vi "io.interface.serial.vi"(0 "IoConf in":T1={"ADDR"=0, "Label"="", "Type"=enum."DI", "Mode"=enum."RIO", "Value"="", "Tags"="", "calibration"=[]} {"calibration"."Y" format="%#.3f"; "calibration"."X" format="%#.3f"; "ADDR" format="%04d"}, 1 "Caller":string, 5 "Output State":variant, 7 "record filename.* (disabled if empty)":string, 9 "current time":timestamp, 11 "error in (no error)":errorcluster, 12 "Save to IO Reg(T)":bool=TRUE) -> (3 "DI":bool[](array[boolean]), 4 "IoConf out":T1={"ADDR"=0, "Label"="", "Type"=enum."DI", "Mode"=enum."RIO", "Value"="", "Tags"="", "calibration"=[]} {"calibration"."Y" format="%#.3f"; "calibration"."X" format="%#.3f"; "ADDR" format="%04d"}, 6 "IN (calib)":dbl, 10 "IN (uncalib)":u16, 14 "Operation Time ms":u32, 15 "error out":errorcluster)   [LabVIEW 2024]
uses:
  controls/IONode.ctl
  controls/type.address.ctl
  controls/enum.io.type.ctl
  controls/enum.io.mode.ctl
  controls/typeXyPoint.ctl
  controls/enum.io-interface.ctl
  controls/enumVarCtrlIO.ctl
  controls/cluster-com-log.ctl
  controls/enum-com-log.ctl
  Polymorphics/io.command-builder.DO.vi
  Polymorphics/io.command-builder.AI.vi
  Polymorphics/io.command-builder.DI.vi
  globals/globals-engine.vi
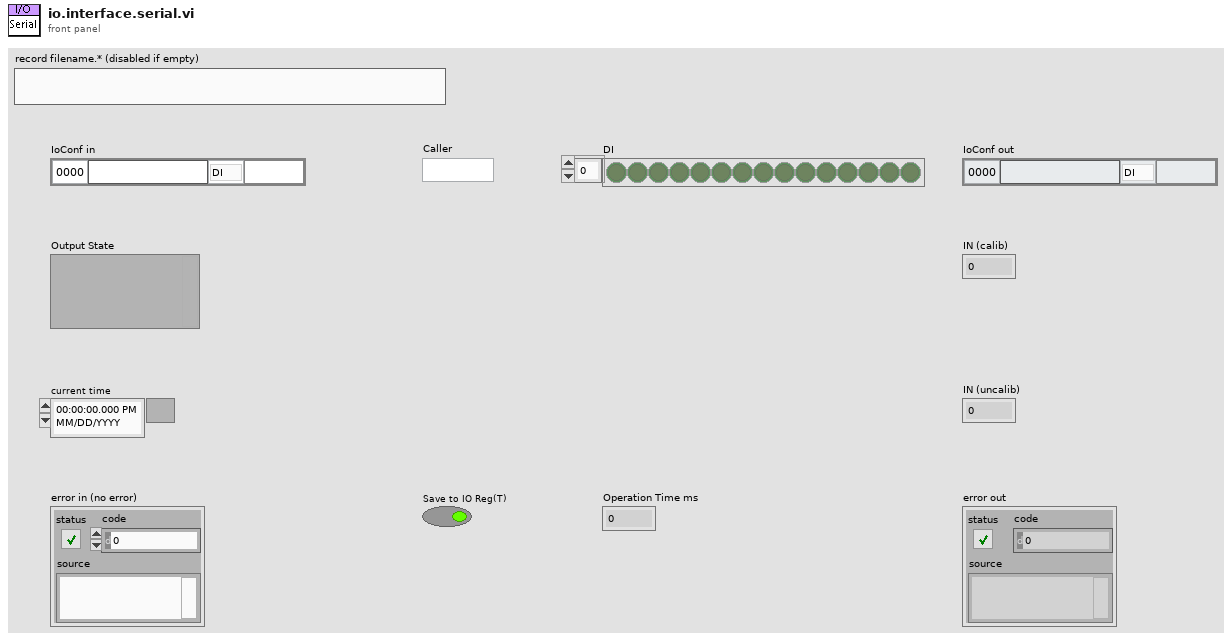
[diagram p1: front panel]
types:
  T1 = typedef "IONode.ctl" = cluster{"ADDR":T2, "Label":string, "Type":T3, "Mode":T4, "Value":string, "Tags":string, "calibration":T5[]}
  T2 = typedef "type.address.ctl" = u16
  T3 = typedef "enum.io.type.ctl" = enum16{"Type", "DI", "DO", "AI", "AO", "VL", "BUF"}
  T4 = typedef "enum.io.mode.ctl" = enum16{"Mode", "RIO", "SIM"}
  T5 = typedef "typeXyPoint.ctl" = cluster{"X":dbl, "Y":dbl}
  T6 = typedef "enum.io-interface.ctl" = enum16{"IO_VISA_WR-RD", "IO_VISA_OPEN", "IO_VISA_CLOSE", "IO_VISA_CLEAR"}
  T7 = typedef "enumVarCtrlIO.ctl" = enum16{"IO Get By Key", "IO List Configs", "IO Add By Key", "IO Modify Value By Key", "IO Modify Calib By Key", "IO Modify ADDR By Key", "IO Modify Mode By Key", "IO Modify Type By Key", "IO Modify Name By Key", "IO Remove By Key", "IO Remove All"}
  T8 = typedef "typeEnv.ctl" = enum16{"ENV.PRODUCTION", "ENV.TEST.NO-HW", "ENV.TEST.SINGLE-01", "ENV.TEST.SINGLE-02", "ENV.TEST.SINGLE-02 AI 0", "ENV.TEST.SINGLE-03"}
  T9 = typedef "cluster-com-log.ctl" = cluster{"Caller":string, "IOnode":T1, "error":errorcluster, "dports":bool[], "AIN (calib)":dbl, "AIN (raw)":u16, "Times Stamp":timestamp, "Record File Path":path, "Visa Data":string}
  T10 = typedef "enum-com-log.ctl" = enum16{"REC.NO_OP", "REC.INIT", "REC.EXIT", "REC.SERIAL", "REC.IO", "REC.FETCH", "REC.OPEN-FILE", "REC.REOPEN-FILE"}
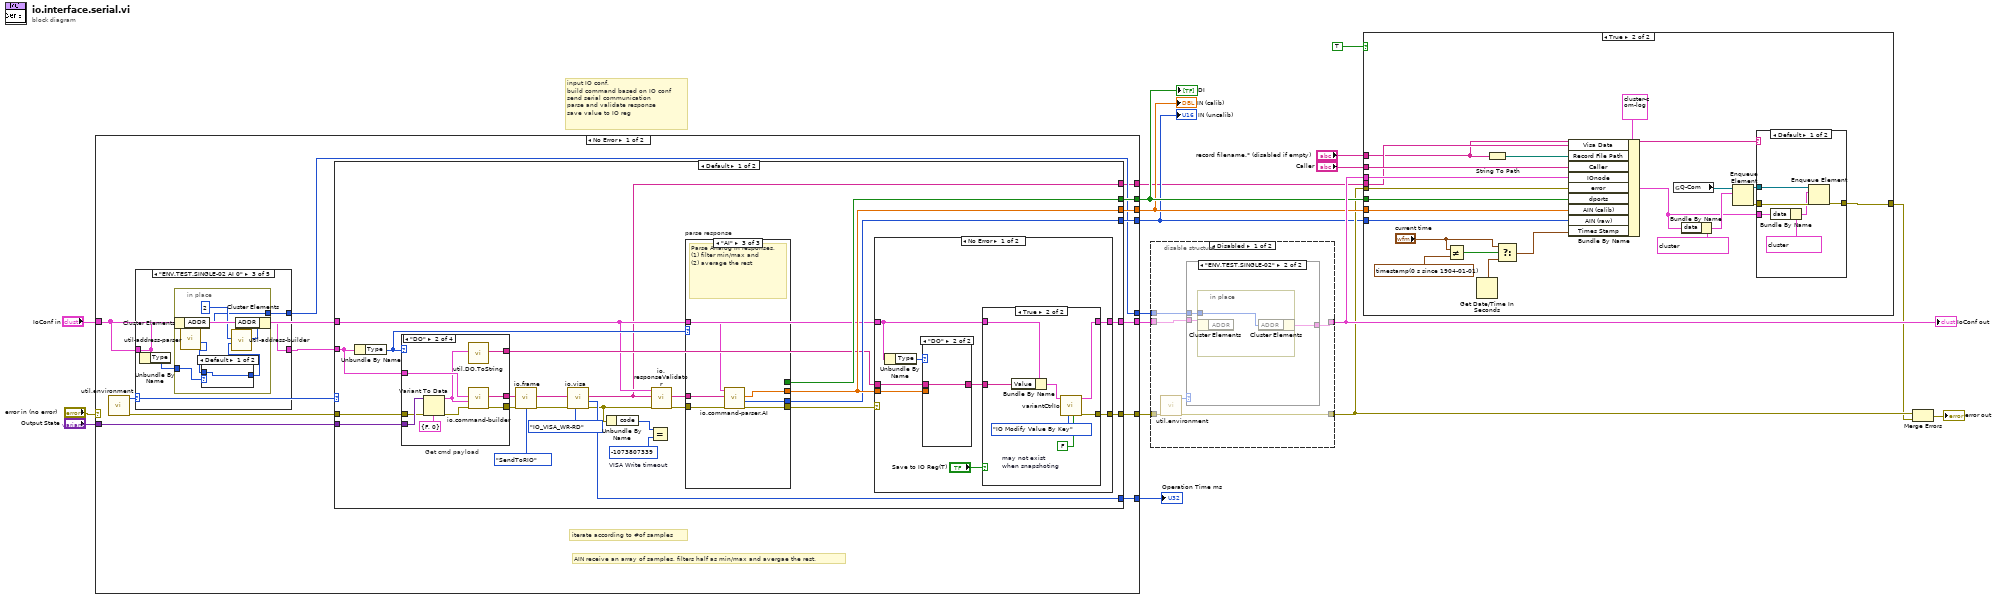
[diagram p0: block diagram]
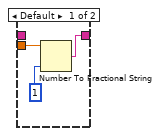
[diagram p6: hidden frame]
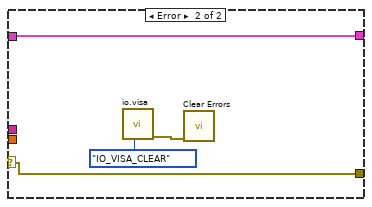
[diagram p8: hidden frame]
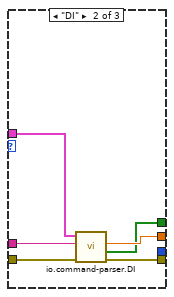
[diagram p10: hidden frame]
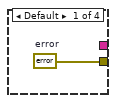
[diagram p11: hidden frame]
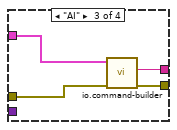
[diagram p12: hidden frame]
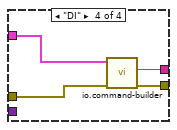
[diagram p13: hidden frame]
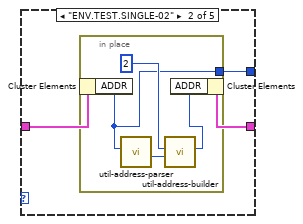
[diagram p16: hidden frame]
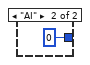
[diagram p17: hidden frame]
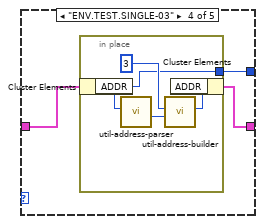
[diagram p18: hidden frame]
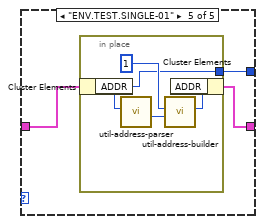
[diagram p19: hidden frame]
diagram:
  # "input IO conf, \nbuild command based on IO conf\nsend serial communication\nparse and validate response\nsave value to IO reg"
  n1 = case shown="No Error" "error in (no error)" {
    selector: "error in (no error)" -> [_ w148]
    tunnel: [w31 _] -> w18
    tunnel: [w30 w148] -> w14
    tunnel: [w29 _] -> w7
    tunnel: [w28 _] -> w4
    tunnel: [w27 _] -> w8
    tunnel: [w26 w147] -> w13
    tunnel: "Output State" -> [w25 _]
    tunnel: "IoConf in" -> [w20 w147]
    tunnel: [w22 _] -> w12
    tunnel: [w19 _] -> w1
    frame No Error {
      # "AIN receive an array of samples, filters half as min/max and avergae the rest."
      # "iterate according to #of samples"
      n2 = call "util.environment.vi"() -> ("error out"=w24:errorcluster, "ENV out"=w21:T8)  [unwired: 10 in]
      n3 = case shown="\"ENV.TEST.SINGLE-02 AI 0\"" w21 {
        tunnel: [w113 w115 w124 w134 w141] -> w23
        tunnel: w20 -> [w113 w116 w122 w135 w142]
        tunnel: [_ w114 w123 w133 w140] -> w22
        frame Default {
        }
        frame "ENV.TEST.SINGLE-02" {
          n4 = in-place {
            in-place-border: [w117] -> w114
            n5 = in-place-cluster #1(w116) -> ("ADDR"=w117:T2)
            n6 = call "util-address-parser.vi"("ADDR 2"=w117) -> ("Channel"=w120:u8)  [unwired: 9 in, 1 out]
            n7 = call "util-address-builder.vi"("Channel"=w120, "Device"=T2 2 ("ADDR")) -> ("ADDR"=w119:T2)  [unwired: 9 in]
            n8 = in-place-cluster #1("ADDR"=w119) -> (w115:T1)
          }
        }
        frame "ENV.TEST.SINGLE-02 AI 0" {
          n9 = Unbundle By Name(w122) -> ("Type"=w121:T3)
          n10 = in-place {
            in-place-border: [w128] -> w123
            in-place-border: w121 -> [w127]
            n11 = in-place-cluster #2(w122) -> ("ADDR"=w128:T2)
            n12 = call "util-address-parser.vi"("ADDR 2"=w128) -> ("Channel"=w126:u8)  [unwired: 9 in, 1 out]
            n13 = case shown="Default" w127 {
              tunnel: [w131 u8 0 ("Channel")] -> w125
              tunnel: w126 -> [w131 _]
              frame Default {
              }
              frame "AI" {
              }
            }
            n14 = call "util-address-builder.vi"("Channel"=w125, "Device"=T2 2 ("ADDR")) -> ("ADDR"=w130:T2)  [unwired: 9 in]
            n15 = in-place-cluster #2("ADDR"=w130) -> (w124:T1)
          }
        }
        frame "ENV.TEST.SINGLE-03" {
          n16 = in-place {
            in-place-border: [w136] -> w133
            n17 = in-place-cluster #3(w135) -> ("ADDR"=w136:T2)
            n18 = call "util-address-parser.vi"("ADDR 2"=w136) -> ("Channel"=w139:u8)  [unwired: 9 in, 1 out]
            n19 = call "util-address-builder.vi"("Channel"=w139, "Device"=T2 3 ("ADDR")) -> ("ADDR"=w138:T2)  [unwired: 9 in]
            n20 = in-place-cluster #3("ADDR"=w138) -> (w134:T1)
          }
        }
        frame "ENV.TEST.SINGLE-01" {
          n21 = in-place {
            in-place-border: [w143] -> w140
            n22 = in-place-cluster #4(w142) -> ("ADDR"=w143:T2)
            n23 = call "util-address-parser.vi"("ADDR 2"=w143) -> ("Channel"=w146:u8)  [unwired: 9 in, 1 out]
            n24 = call "util-address-builder.vi"("Channel"=w146, "Device"=T2 1 ("ADDR")) -> ("ADDR"=w145:T2)  [unwired: 9 in]
            n25 = in-place-cluster #4("ADDR"=w145) -> (w141:T1)
          }
        }
      }
      n26 = case shown="Default" w21 {
        tunnel: [w56 _] -> w31
        tunnel: [w55 _] -> w30
        tunnel: [w54 _] -> w29
        tunnel: [w53 _] -> w28
        tunnel: [w52 _] -> w27
        tunnel: [w51 w112] -> w26
        tunnel: w25 -> [w50 _]
        tunnel: w24 -> [w49 _]
        tunnel: w23 -> [w41 w112]
        tunnel: w20 -> [w34 _]
        tunnel: [w33 _] -> w19
        frame Default {
          w37 = -1073807339  # VISA Write timeout
          n27 = Unbundle By Name(w41) -> ("Type"=w43:T3)
          n28 = case "Get cmd payload" shown="\"DO\"" w43 {
            tunnel: w41 -> [_ w101 w104 w108]
            tunnel: [_ w103 w107 w111] -> w44
            tunnel: [w94 w102 w106 w110] -> w45
            tunnel: w49 -> [_ w97 w105 w109]
            tunnel: w50 -> [_ w99 _ _]
            tunnel: [_ w95 _ _] -> w40
            frame Default {
              w94 = errorcluster {"status"=TRUE, "code"=-1, "source"="Command Error"}  # error
            }
            frame "DO" {
              n29 = Variant To Data(error in=w97, type=cluster{"state":bool, "timeoutSeconds":u16} {"state"=FALSE, "timeoutSeconds"=0}, Variant=w99) -> (data=w96:cluster{"state":bool, "timeoutSeconds":u16}, error out=w98:errorcluster)
              n30 = call "util.DO.ToString.vi"("output cluster"=w96) -> ("initial string"=w95:string)  [unwired: 9 in, 1 out]
              n31 = call-poly "io.command-builder.vi"("error in"=w98, "parsed dout state"=w96, "IoConf in"=w101) -> ("error out"=w102:errorcluster, "Frameless Command"=w103:string)  [unwired: 7 in]
            }
            frame "AI" {
              n32 = call-poly "io.command-builder.vi"("error in"=w105, "IoConf in"=w104) -> ("error out"=w106:errorcluster, "Generated Command"=w107:string)  [unwired: 8 in]
            }
            frame "DI" {
              n33 = call-poly "io.command-builder.vi"("error in"=w109, "IoConf in"=w108) -> ("error out"=w110:errorcluster, "Generated Command"=w111:string)  [unwired: 8 in]
            }
          }
          n34 = call "io.frame.vi"("error in"=w45, "Direction (To RIO)"=enum16{"SendToRIO", "ReceiveFromRio"}."SendToRIO", "Frameless Command"=w44) -> ("error out"=w46:errorcluster, "Framed Command"=w47:string)  [unwired: 7 in]
          n35 = call "io.visa.vi"("operation in (wr-rd)"=enum.io-interface."IO_VISA_WR-RD" ("operation"), "error in (no error)"=w46, "write buffer"=w47) -> ("error out"=w39:errorcluster, "delta"=w56:u32, "read buffer"=w33:string)  [unwired: 5 in, 1 out]
          n36 = Unbundle By Name(w39) -> ("code"=w38:i32)
          n37 = Equal?(x=w38, y=w37) -> ()  [unwired: 1 out]
          n38 = call "io.responseValidator.vi"("error in"=w39, "ResponsToValidate in"=w33, "IoConf in 2"=w34) -> ("error out"=w35:errorcluster, "Data out"=w32:string)  [unwired: 7 in]
          n39 = case "parse response" shown="\"AI\"" w43 {
            tunnel: w32 -> [_ w83 w93]
            tunnel: [w81 w87 w92] -> w42
            tunnel: [_ w86 w91] -> w54
            tunnel: w34 -> [_ w82 w90]
            tunnel: [_ _ w89] -> w53
            tunnel: [_ w85 _] -> w52
            tunnel: w35 -> [w81 w84 w88]
            frame Default {
            }
            frame "DI" {
              n40 = call "io.command-parser.DI.vi"("error in (no error)"=w84, "Reponse in"=w83, "IoConf out"=w82) -> ("error out"=w87:errorcluster, "dports"=w85:bool[], "DI out"=w86:dbl)  [unwired: 6 in]
            }
            frame "AI" {
              # "Parse Analog In responses,  (1) filter min/max and \n(2) average the rest"
              n41 = call "io.command-parser.AI.vi"("error in"=w88, "Reponse in"=w93, "IoConf in"=w90) -> ("error out"=w92:errorcluster, "AI uncalib out"=w89:u16, "AI out"=w91:dbl)  [unwired: 6 in]
            }
          }
          n42 = case shown="No Error" w42 {
            selector: w42 -> [_ w77]
            tunnel: [w64 w77] -> w55
            tunnel: w54 -> [w63 _]
            tunnel: [w62 w80] -> w51
            tunnel: w34 -> [w59 w80]
            tunnel: w40 -> [w58 _]
            frame No Error {
              n43 = Unbundle By Name(w59) -> ("Type"=w60:T3)
              n44 = case shown="\"DO\"" w60 {
                tunnel: [w67 w68] -> w61
                tunnel: w63 -> [w66 _]
                tunnel: w58 -> [_ w68]
                frame Default {
                  n45 = Number To Fractional String(number=w66, precision (6)=i16 1) -> (F-format string=w67:string)  [unwired: 2 in]
                }
                frame "DO" {
                }
              }
              n46 = case shown="True" "Save to IO Reg(T)" {
                tunnel: w61 -> [_ w76]
                tunnel: [_ w74] -> w64
                tunnel: [w69 w70] -> w62
                tunnel: w59 -> [w69 w72]
                frame False {
                }
                frame True {
                  w73 = FALSE  # may not exist when snapshoting
                  n47 = Bundle By Name(cluster=w72, "Value"=w76) -> (w71:T1)
                  n48 = call "variantCtrlIo.vi"("isRequired (T)"=w73, "menu (Get Param)"=enumVarCtrlIO."IO Modify Value By Key" ("menu (get)"), "IOnode in"=w71) -> ("error out"=w74:errorcluster, "IOnode out"=w70:T1)  [unwired: 4 in, 3 out]
                }
              }
            }
            frame Error {
              n49 = call "io.visa.vi"("operation in (wr-rd)"=enum.io-interface."IO_VISA_CLEAR") -> ("error out"=w78:errorcluster)  [unwired: 7 in, 3 out]
              n50 = call <vilib>:"Clear Errors.vi"("error in (no error)"=w78) -> ()  [unwired: 5 in, 2 out]
            }
          }
        }
        frame "ENV.TEST.NO-HW" {
        }
      }
    }
    frame Error {
    }
  }
  "Operation Time ms" <- w18
  "IN (calib)" <- w7
  "IN (uncalib)" <- w4
  "DI" <- w8
  n51 = disable-structure shown="Disabled" {
    disable-tunnel: w14 -> [w154 w160]
    disable-tunnel: w13 -> [w152 w161]
    disable-tunnel: w12 -> [w151 _]
    disable-tunnel: [w150 w161] -> w10
    disable-tunnel: [w149 w160] -> w6
    frame Disabled {
      n52 = call "util.environment.vi"("error in"=w154) -> ("error out"=w149:errorcluster, "ENV out"=w153:T8)  [unwired: 9 in]
      n53 = case shown="\"ENV.TEST.SINGLE-02\"" w153 {
        tunnel: w152 -> [w155 w158]
        tunnel: [w155 w157] -> w150
        tunnel: w151 -> [_ w156]
        frame Default {
        }
        frame "ENV.TEST.SINGLE-02" {
          n54 = in-place {
            in-place-border: w156 -> [w159]
            n55 = in-place-cluster #5(w158) -> ()  [unwired: 1 out]
            n56 = in-place-cluster #5("ADDR"=w159) -> (w157:T1)
          }
        }
      }
    }
    frame Enabled {
    }
  }
  "IoConf out" <- w10
  n57 = case shown="True" TRUE {
    tunnel: "Caller" -> [_ w183]
    tunnel: w10 -> [_ w182]
    tunnel: w8 -> [_ w181]
    tunnel: w7 -> [_ w180]
    tunnel: w6 -> [_ w179]
    tunnel: w4 -> [_ w178]
    tunnel: [_ w165] -> w3
    tunnel: "record filename.* (disabled if empty)" -> [_ w162]
    tunnel: w1 -> [_ w168]
    frame False {
    }
    frame True {
      n58 = Not Equal?(x="current time", y=timestamp(0 s since 1904-01-01)) -> (x != y?=w173:bool)
      n59 = Get Date/Time In Seconds() -> (seconds since 1Jan1904=w176:timestamp)
      n60 = String To Path(string=w162) -> (path=w170:path)
      n61 = Select(t="current time", s=w173, f=w176) -> (s? t:f=w171:timestamp)
      n62 = Bundle By Name(cluster=T9 {"Caller"="", "IOnode"={"ADDR"=0, "Label"="Name", "Type"=enum."DI", "Mode"=enum."RIO", "Value"="Value", "Tags"="Tags", "calibration"=[]}, "error"={"status"=FALSE, "code"=0, "source"=""}, "dports"=[], "AIN (calib)"=0.0, "AIN (raw)"=0, "Times Stamp"=timestamp(0 s since 1904-01-01), "Record File Path"=path "", "Visa Data"=""} ("input cluster"), "Visa Data"=w168, "Record File Path"=w170, "Caller"=w183, "IOnode"=w182, "error"=w179, "dports"=w181, "AIN (calib)"=w180, "AIN (raw)"=w178, "Times Stamp"=w171) -> (w163:T9)
      n63 = global read "globals-engine.vi" "Q-Com"() -> (w169:refnum<queue>)
      n64 = Bundle By Name(cluster=cluster{"data":variant, "Enum":T10} {"data"=variant, "Enum"=enum."REC.SERIAL"} ("procQ"), "data"=w163) -> (w164:cluster{"data":variant, "Enum":T10})
      n65 = Enqueue Element(queue=w169, element=w164) -> (queue out=w167:refnum<queue>, error out=w166:errorcluster)  [unwired: 2 in, 1 out]
      n66 = case shown="Default" w162 {
        tunnel: w167 -> [w189 _]
        tunnel: w166 -> [w188 w190]
        tunnel: [w187 w190] -> w165
        tunnel: w163 -> [w186 _]
        frame Default {
          n67 = Bundle By Name(cluster=cluster{"data":variant, "Enum":T10} {"data"=variant, "Enum"=enum."REC.IO"} ("procQ"), "data"=w186) -> (w185:cluster{"data":variant, "Enum":T10})
          n68 = Enqueue Element(queue=w189, element=w185, error in (no error)=w188) -> (error out=w187:errorcluster)  [unwired: 1 in, 2 out]
        }
        frame "" {
          # "empty filename - skip io record"
        }
      }
    }
  }
  n69 = Merge Errors(w6, w3) -> (→"error out":errorcluster)
